vi "Form Monotonically Increasing Name.vi"(8 "error in (no error)":errorcluster, 10 "index":i32, 11 "Desired Name":string) -> (0 "error out":errorcluster, 2 "next index":i32, 3 "Next Candidate Name":string)   [LabVIEW 2020, in "Routing and Faulting System Explorer.lvlib"]
uses:
  Routing and Faulting System Explorer.lvlib
  <vilib>/regexp/Match Regular Expression.xnode
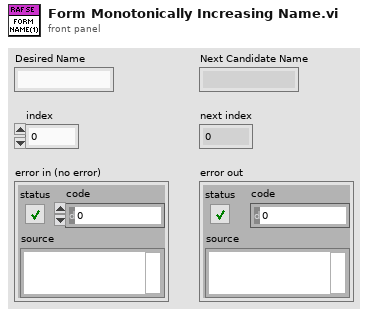
[diagram p1: front panel]
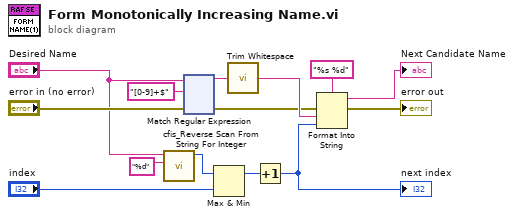
[diagram p0: block diagram]
diagram:
  n1 = call <vilib>:"cfis_Reverse Scan From String For Integer.vi"("format string"="%d", "input string"="Desired Name") -> ("Extracted integer"=w2:i32)  [unwired: 9 in]
  n2 = xnode "Match Regular Expression"("input string"="Desired Name", "regular expression"="[0-9]+$", "error in"="error in (no error)") -> ("before match"=w12:string, "error out"=w10:errorcluster)  [unwired: 3 in, 3 out]
  n3 = Max & Min(x=w2, y="index") -> (max(x,y)=w6:i32)  [unwired: 1 out]
  n4 = call <vilib>:"Trim Whitespace.vi"("string"=w12) -> ("trimmed string"=w13:string)  [unwired: 1 in]
  n5 = Increment(x=w6) -> (x+1=w14:i32)
  "next index" <- w14
  n6 = Format Into String(format string="%s %d", error in=w10, w13, w14) -> (resulting string=→"Next Candidate Name":string, error out=→"error out":errorcluster)  [unwired: 1 in]
